vi "When Read Double.vi"(0 "error out":errorcluster, 1 "value":dbl, 11 "Configuration In":refnum<class "Mock Configuration.lvclass">) -> (3 "Configuration Out":refnum<class "Mock Configuration.lvclass">)   [LabVIEW 2020, in "Mock Configuration.lvclass"]
doc: "High-level function for reading configuration file data from process class. If the specified key is not present, it is added with the configured default value."
uses:
  Mock Configuration.lvclass
  C:/Program Files (x86)/National Instruments/LabVIEW 2020/vi.lib/Astemes/LMock/Mock.lvclass
  <vilib>/Astemes/LMock/Mock.lvclass
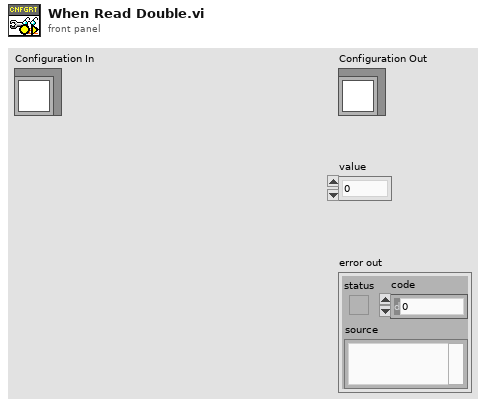
[diagram p1: front panel]
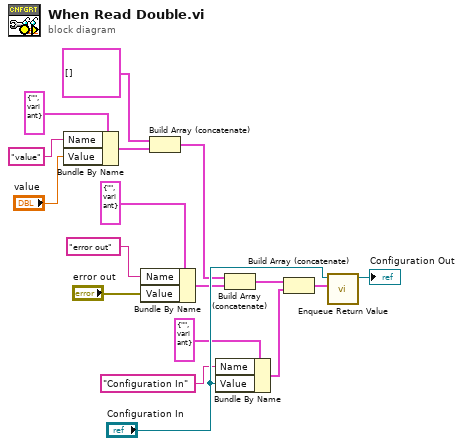
[diagram p0: block diagram]
diagram:
  n1 = Bundle By Name(cluster=cluster{"Name":string, "Value":variant} {"Name"="", "Value"=variant} ("element"), "Name"="value", "Value"="value") -> (w5:cluster{"Name":string, "Value":variant})
  n2 = Bundle By Name(cluster=cluster{"Name":string, "Value":variant} {"Name"="", "Value"=variant} ("element"), "Name"="error out", "Value"="error out") -> (w3:cluster{"Name":string, "Value":variant})
  n3 = Build Array (concatenate)(cluster{"Name":string, "Value":variant}[] [] ("Control Values"), w5) -> (w10:cluster{"Name":string, "Value":variant}[])
  n4 = Bundle By Name(cluster=cluster{"Name":string, "Value":variant} {"Name"="", "Value"=variant} ("element"), "Name"="Configuration In", "Value"="Configuration In") -> (w1:cluster{"Name":string, "Value":variant})
  n5 = Build Array (concatenate)(w10, w3) -> (w13:cluster{"Name":string, "Value":variant}[])
  n6 = Build Array (concatenate)(w13, w1) -> (w15:cluster{"Name":string, "Value":variant}[])
  n7 = call <vilib>:"Enqueue Return Value.vi"("Indicator Values"=w15, "Mock In"="Configuration In") -> ("Mock Out"=→"Configuration Out":refnum<class "Mock Configuration.lvclass">)  [unwired: 8 in, 1 out]
